vi "Get.vi"(11 "Name":string) -> (1 "Remove/Found":bool, 2 "DebugTracerOut":refnum<class "DebugTraceHandle.lvclass">)   [LabVIEW 2024, in "DebugTraceSingleton.lvlib"]
uses:
  DebugTraceSingleton.lvlib
  DebugTraceHandle/DebugTraceHandle.lvclass
  Command.ctl
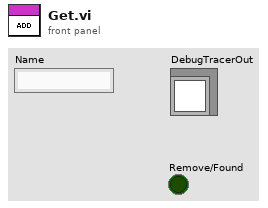
[diagram p1: front panel]
types:
  T1 = typedef "DebugTraceSingleton.lvlib/Command.ctl" = enum16{"Add", "Remove", "Get", "GetAll"}
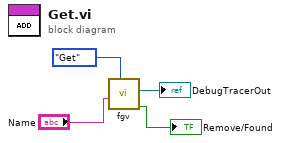
[diagram p0: block diagram]
diagram:
  n1 = call "fgv.vi"("Command"=Command."Get", "Name"="Name") -> ("Remove/Found"=→"Remove/Found":bool, "DebugTracerOut"=→"DebugTracerOut":refnum<class "DebugTraceHandle.lvclass">)  [unwired: 7 in, 1 out]
